vi "Associate Instruments to Paths.vi"(0 "Scalar Path Group in":refnum<class "Scalar Path Group.lvclass">, 5 "TSM Context":T1, 11 "error in (no error)":errorcluster) -> (4 "Scalar Path Group out":refnum<class "Scalar Path Group.lvclass">, 15 "error out":errorcluster)   [LabVIEW 2023, in "RFFixtureCharact.Public.lvlib" / "Scalar Path Group.lvclass"]
uses:
  Scalar Path Group.lvclass
  <vilib>/NI_TestStand_SemiconductorModule/NI_TestStand_Semiconductor_Module.lvlibp/PinMap/General/SemiconductorModuleContext.ctl
  <vilib>/NI_TestStand_SemiconductorModule/NI_TestStand_Semiconductor_Module.lvlibp
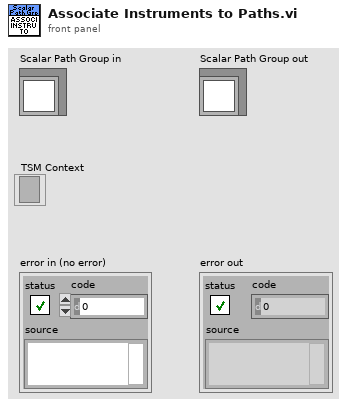
[diagram p1: front panel]
types:
  T1 = typedef "NI_TestStand_Semiconductor_Module.lvlibp/SemiconductorModuleContext.ctl" = refnum<k7>
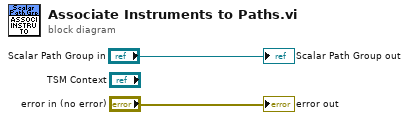
[diagram p0: block diagram]
diagram:
  "error out" <- "error in (no error)"
  "Scalar Path Group out" <- "Scalar Path Group in"
